vi "PwrMtr_U2k_MatchIDNStr.vi"(8 "error in":errorcluster, 10 "IDNStr":string) -> (0 "error out":errorcluster, 2 "IDN match":bool, 3 "ClassLibraryFile":path)   [LabVIEW 2014]
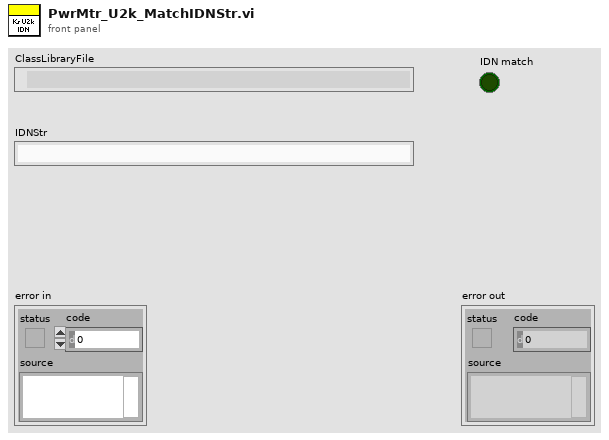
[diagram p1: front panel]
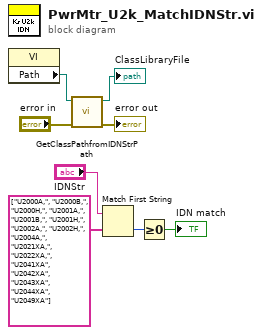
[diagram p0: block diagram]
diagram:
  n1 = property class="VI"() -> ("Path"=w5:path)  [unwired: 2 in, 2 out]
  n2 = call "GetClassPathfromIDNStrPath.vi"("error in (no error)"="error in", "Path in"=w5) -> ("error out"=→"error out":errorcluster, "Path out"=→"ClassLibraryFile":path)  [unwired: 8 in]
  n3 = Match First String(2:string[] ["U2000A,", "U2000B,", "U2000H,", "U2001A,", "U2001B,", "U2001H,", "U2002A,", "U2002H,", "U2004A,", "U2021XA,", "U2022XA,", "U2041XA", "U2042XA", "U2043XA", "U2044XA", "U2049XA"] ("string array"), 3:"IDNStr") -> (0:w7:i32)  [unwired: 1 out]
  n4 = Greater Or Equal To 0?(x=w7) -> (x >= 0?=→"IDN match":bool)
